vi "Display_OverlayScoreRGB.vi"(1 "Player":T1, 4 "ActivePixel":T2) -> (15 "Draw":bool, 16 "Red":bool, 17 "Green":bool, 18 "Blue":bool)   [LabVIEW 2018]
uses:
  TypDefs/ActivePixel_Cluster.ctl
  TypDefs/Player_Enum.ctl
  FPGA VGA Graphics/FPGA VGA Library/TypDefs/VGA_Position.ctl
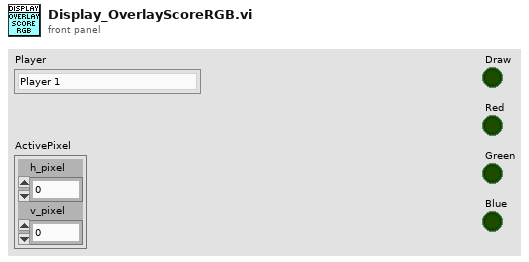
[diagram p1: front panel]
types:
  T1 = typedef "Player_Enum.ctl" = enum16{"Player 1", "Player 2"}
  T2 = typedef "ActivePixel_Cluster.ctl" = cluster{"h_pixel":i16, "v_pixel":i16}
  T3 = typedef "VGA_Position.ctl" = cluster{"h_pixel":i16, "v_pixel":i16}
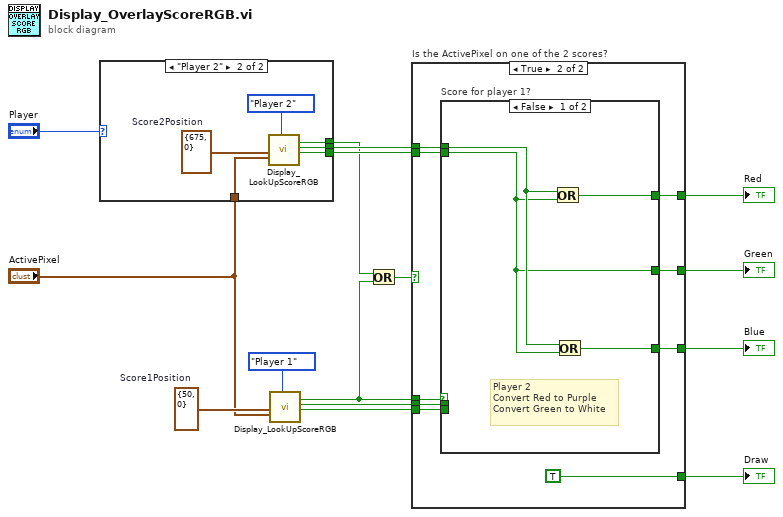
[diagram p0: block diagram]
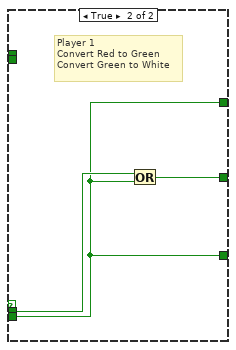
[diagram p4: hidden frame]
diagram:
  w15 = T3 {"h_pixel"=50, "v_pixel"=0}  # Score1Position
  n1 = case shown="\"Player 2\"" "Player" {
    tunnel: "ActivePixel" -> [_ w21]
    tunnel: [_ w19] -> w1
    tunnel: [_ w18] -> w11
    tunnel: [_ w17] -> w10
    frame "Player 1" {
    }
    frame "Player 2" {
      w20 = T3 {"h_pixel"=675, "v_pixel"=0}  # Score2Position
      n2 = call "Display_LookUpScoreRGB.vi"("Position"=w20, "ActivePixel"=w21, "Player"=Player_Enum."Player 2") -> ("Draw"=w19:bool, "Red"=w18:bool, "Green"=w17:bool)  [unwired: 13 in, 1 out]
    }
  }
  n3 = call "Display_LookUpScoreRGB.vi"("Position"=w15, "ActivePixel"="ActivePixel", "Player"=Player_Enum."Player 1") -> ("Draw"=w7:bool, "Red"=w9:bool, "Green"=w8:bool)  [unwired: 13 in, 1 out]
  n4 = Or(x=w1, y=w7) -> (x .or. y?=w12:bool)
  n5 = case "Is the ActivePixel on one of the 2 scores?" shown="True" w12 {
    tunnel: w7 -> [_ w30]
    tunnel: w11 -> [_ w29]
    tunnel: w10 -> [_ w28]
    tunnel: w9 -> [_ w27]
    tunnel: w8 -> [_ w26]
    tunnel: [_ TRUE] -> w6
    tunnel: [_ w24] -> w5
    tunnel: [_ w23] -> w4
    tunnel: [_ w22] -> w3
    frame False {
    }
    frame True {
      n6 = case "Score for player 1?" shown="False" w30 {
        tunnel: w29 -> [w34 _]
        tunnel: w28 -> [w31 _]
        tunnel: w27 -> [_ w36]
        tunnel: w26 -> [_ w35]
        tunnel: [w31 w37] -> w24
        tunnel: [w32 w35] -> w23
        tunnel: [w33 w35] -> w22
        frame False {
          # "Player 2\nConvert Red to Purple\nConvert Green to White"
          n7 = Or(x=w34, y=w31) -> (x .or. y?=w32:bool)
          n8 = Or(x=w34, y=w31) -> (x .or. y?=w33:bool)
        }
        frame True {
          # "Player 1\nConvert Red to Green\nConvert Green to White"
          n9 = Or(x=w36, y=w35) -> (x .or. y?=w37:bool)
        }
      }
    }
  }
  "Red" <- w4
  "Green" <- w5
  "Blue" <- w3
  "Draw" <- w6
